vi "start.vi"(8 "error in (no error)":errorcluster, 11 "ProEM_WinX32 in":refnum<class "ProEM_WinX32.lvclass">) -> (0 "error out":errorcluster, 3 "ProEM_WinX32 out":refnum<class "ProEM_WinX32.lvclass">)   [LabVIEW 2009, in "Hardware.lvlib" / "Channels.lvlib" / "ProEM_WinX32.lvclass"]
uses:
  ProEM_WinX32.lvclass
  ProEM_WinX32.lvclass/ProEM_WinX32.ctl
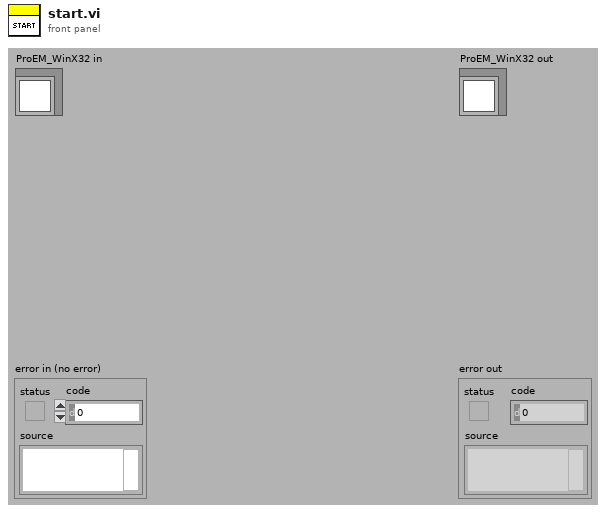
[diagram p1: front panel]
types:
  T1 = typedef "WINX32 Object Reference.ctl" = refnum<k1>
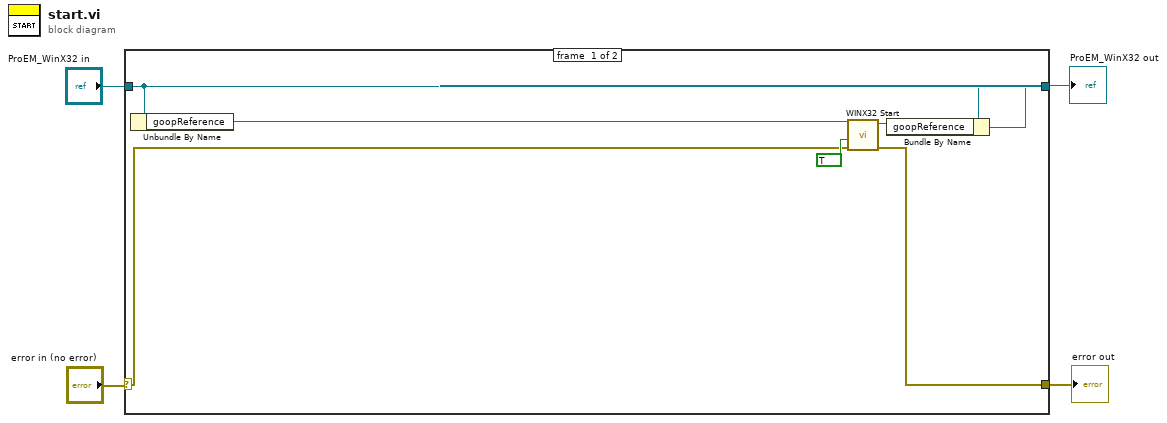
[diagram p0: block diagram]
diagram:
  n1 = case shown="No Error" "error in (no error)" {
    selector: "error in (no error)" -> [w5 w12]
    tunnel: [w10 w13] -> w4
    tunnel: "ProEM_WinX32 in" -> [w11 w13]
    tunnel: [w8 w12] -> w1
    frame #0 {
      n2 = Unbundle By Name(w11) -> ("goopReference"=w6:T1)
      n3 = call <instrlib>:"WINX32 Start.vi"("error in (no error)"=w5, "Camera Active"=TRUE, "reference"=w6) -> ("error out"=w8:errorcluster, "duplicate reference"=w9:T1)  [unwired: 7 in]
      n4 = Bundle By Name(cluster=w11, "goopReference"=w9) -> (w10:refnum<class "ProEM_WinX32.lvclass">)
    }
    frame #1 {
    }
  }
  "error out" <- w1
  "ProEM_WinX32 out" <- w4
